vi "FVI_Manette_Process.vi"(2 "Axe R Y":dbl, 5 "Axe L Y":dbl, 6 "POV":dbl, 7 "Axe R X":dbl, 9 "Rtrigger":dbl, 11 "Axe L X":dbl) -> (1 "Correction angle":dbl, 4 "SwerveDrive":T1)   [LabVIEW 2018]
uses:
  SwerveDrive.ctl
  MyGlobal.vi
panel:
  in  "TD_SwerveDrive":T1
  out "arctan(x)":dbl
  out "x/y":dbl
  out "y < 0":bool
  out "x < 0":bool
  out "error out":errorcluster
  in  "error in (no error)":errorcluster
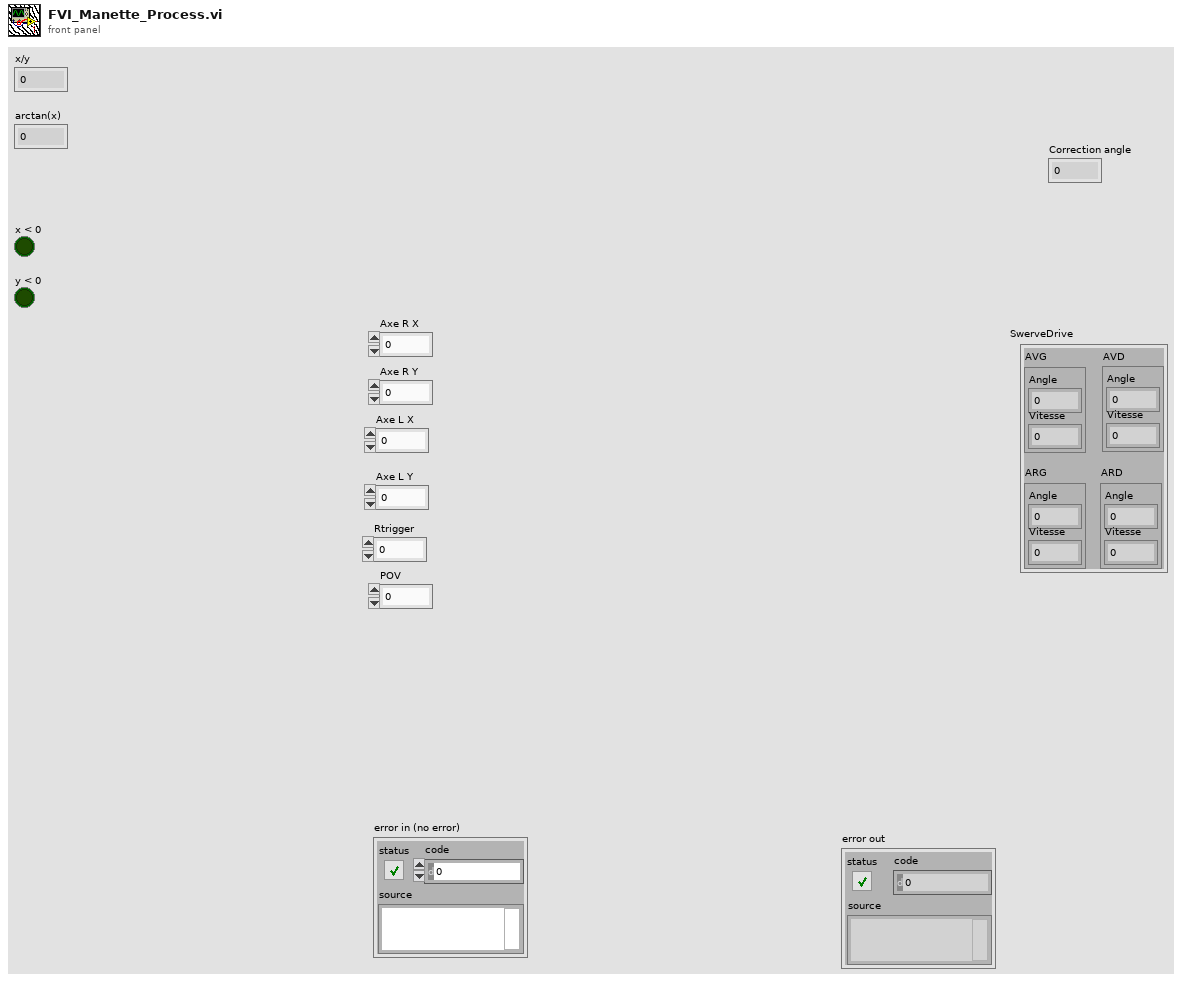
[diagram p1: front panel]
types:
  T1 = typedef "SwerveDrive.ctl" = cluster{"AVD":cluster{"Angle":dbl, "Vitesse":dbl}, "AVG":cluster{"Angle":dbl, "Vitesse":dbl}, "ARG":cluster{"Angle":dbl, "Vitesse":dbl}, "ARD":cluster{"Angle":dbl, "Vitesse":dbl}}
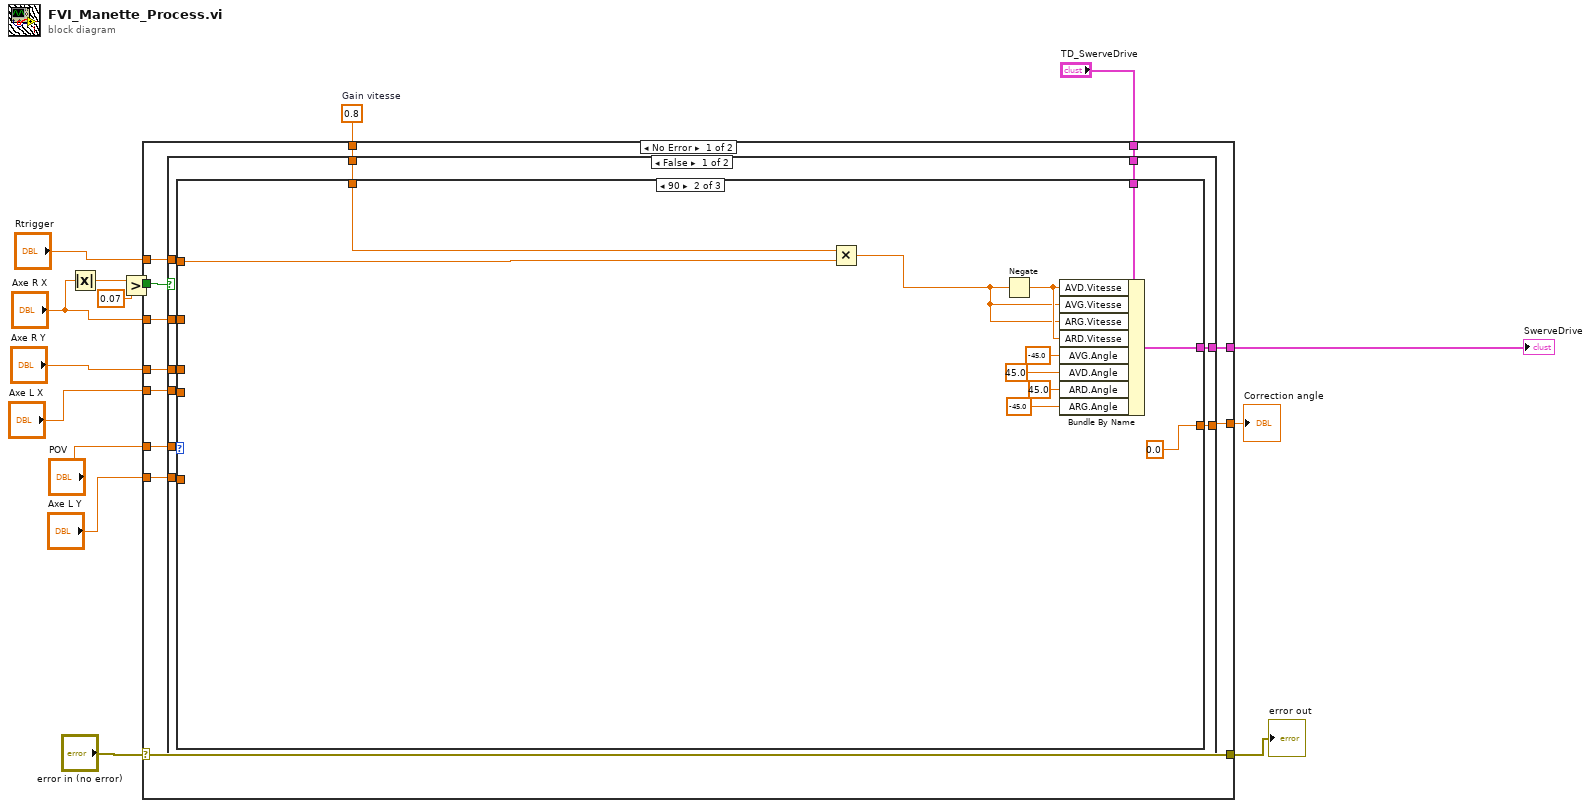
[diagram p0: block diagram]
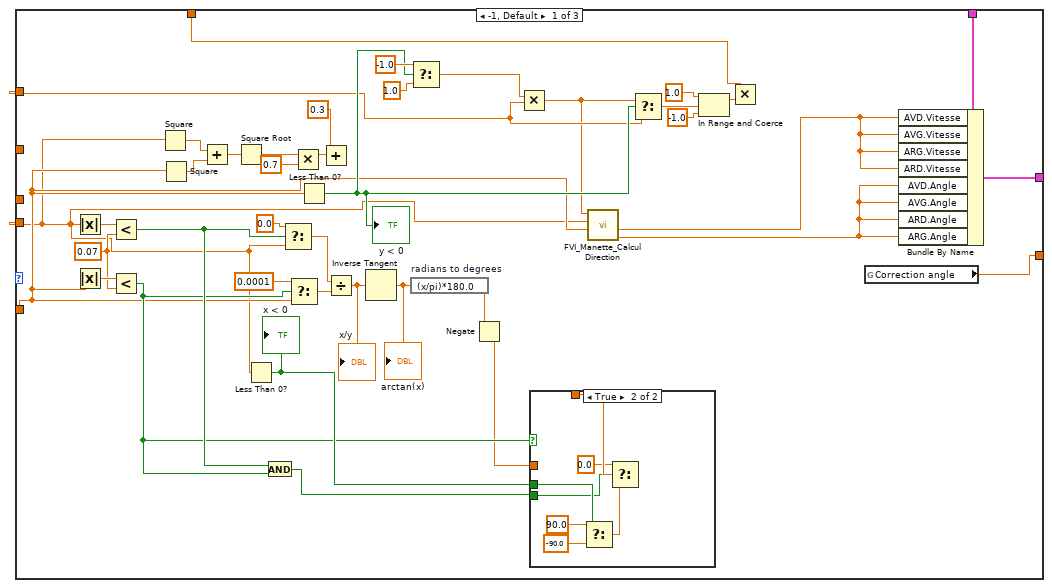
[diagram p2: hidden frame]
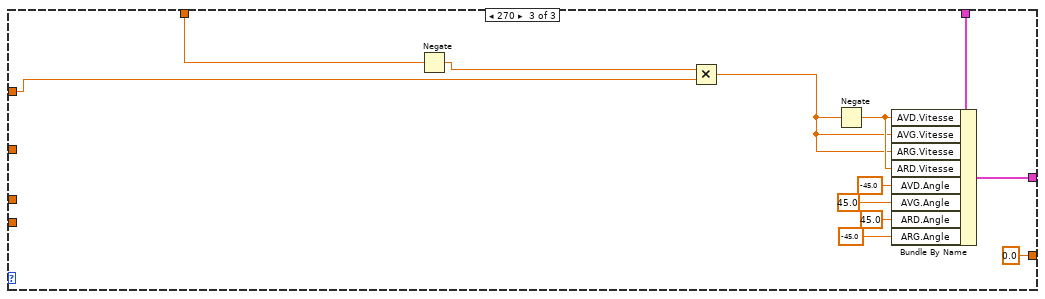
[diagram p4: hidden frame]
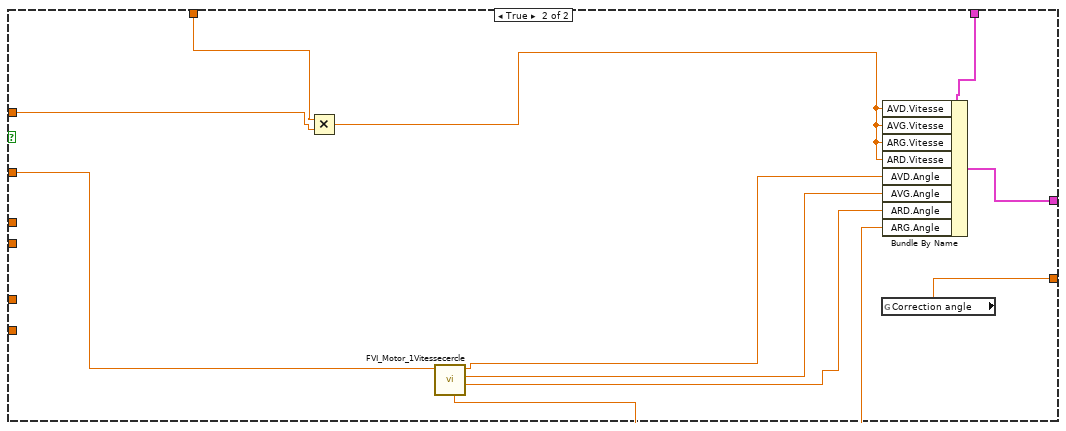
[diagram p5: hidden frame]
diagram:
  w5 = 0.8  # Gain vitesse
  n1 = Absolute Value(x="Axe R X") -> (abs(x)=w10:dbl)
  n2 = Greater?(x=w10, y=0.07 ("t")) -> (0:w8:bool)
  n3 = case shown="No Error" "error in (no error)" {
    selector: "error in (no error)" -> [w26 w121]
    tunnel: "Axe L X" -> [w25 _]
    tunnel: "Axe L Y" -> [w24 _]
    tunnel: [w27 _] -> w1
    tunnel: [w26 w121] -> w13
    tunnel: "Rtrigger" -> [w23 _]
    tunnel: "POV" -> [w22 _]
    tunnel: "Axe R X" -> [w21 _]
    tunnel: "Axe R Y" -> [w20 _]
    tunnel: w8 -> [w19 _]
    tunnel: w5 -> [w18 _]
    tunnel: "TD_SwerveDrive" -> [w17 w120]
    tunnel: [w16 w120] -> w2
    frame No Error {
      n4 = case shown="False" w19 {
        tunnel: [w28 w109] -> w27
        tunnel: w25 -> [w37 _]
        tunnel: w24 -> [w36 _]
        tunnel: w23 -> [w35 w119]
        tunnel: w22 -> [w34 _]
        tunnel: w21 -> [w33 w117]
        tunnel: w20 -> [w32 _]
        tunnel: w18 -> [w31 w118]
        tunnel: w17 -> [w30 w115]
        tunnel: [w29 w114] -> w16
        frame False {
          n5 = case shown="90" w34 {
            tunnel: w37 -> [w41 _ _]
            tunnel: w36 -> [w42 _ _]
            tunnel: w35 -> [w49 w96 w108]
            tunnel: w33 -> [_ _ _]
            tunnel: w32 -> [_ _ _]
            tunnel: w31 -> [w44 w95 w107]
            tunnel: w30 -> [w46 w94 w100]
            tunnel: [w45 w93 w99] -> w29
            tunnel: [w38 0.0 ("Correctiobn angle") 0.0 ("Correctiobn angle")] -> w28
            frame -1, Default {
              w67 = 0.07 ("t")
              n6 = Absolute Value(x=w41) -> (abs(x)=w76:dbl)
              n7 = Absolute Value(x=w42) -> (abs(x)=w77:dbl)
              n8 = Less?(x=w76, y=w67) -> (x < y?=w58:bool)
              n9 = Less?(x=w77, y=w67) -> (x < y?=w57:bool)
              n10 = Square(x=w41) -> (x^2=w54:dbl)
              n11 = Square(x=w42) -> (x^2=w55:dbl)
              n12 = Add(x=w54, y=w55) -> (x+y=w56:dbl)
              n13 = Square Root(x=w56) -> (sqrt(x)=w53:dbl)
              n14 = Less Than 0?(x=w41) -> (x < 0?=w71:bool)
              "x < 0" <- w71
              n15 = And(x=w58, y=w57) -> (x .and. y?=w75:bool)
              n16 = Select(t=0.0, s=w58, f=w41) -> (s? t:f=w63:dbl)
              n17 = Select(t=0.0001, s=w57, f=w42) -> (s? t:f=w61:dbl)
              n18 = Multiply(x=w53, y=0.7) -> (x*y=w51:dbl)
              n19 = Less Than 0?(x=w42) -> (x < 0?=w72:bool)
              "y < 0" <- w72
              n20 = Add(x=0.3, y=w51) -> ()  [unwired: 1 out]
              n21 = Divide(x=w63, y=w61) -> (x/y=w59:dbl)
              "x/y" <- w59
              n22 = Inverse Tangent(1:w59) -> (0:w60:dbl)
              "arctan(x)" <- w60
              n23 = Select(t=-1.0, s=w72, f=1.0) -> (s? t:f=w48:dbl)
              n24 = expression code="(x/pi)*180.0" "radians to degrees"(w60) -> (w69:dbl)
              n25 = Negate(x=w69) -> (-x=w47:dbl)
              n26 = Multiply(x=w48, y=w49) -> (x*y=w40:dbl)
              n27 = case shown="True" w57 {
                tunnel: w47 -> [w78 _]
                tunnel: w71 -> [_ w85]
                tunnel: [w78 w81] -> _
                tunnel: w75 -> [_ w79]
                frame False {
                }
                frame True {
                  n28 = Select(t=90.0, s=w85, f=-90.0) -> (s? t:f=w82:dbl)
                  n29 = Select(t=0.0, s=w79, f=w82) -> (s? t:f=w81:dbl)
                }
              }
              n30 = call "FVI_Manette_Calcul Direction.vi"("Axe L Y"=w42, "Axe L X"=w41, "Gain"=w40) -> ("Angle"=w39:dbl, "Vitesse"=w43:dbl)  [unwired: 5 in, 2 out]
              n31 = Select(t=w40, s=w72, f=w49) -> (s? t:f=w64:dbl)
              n32 = In Range and Coerce(upper limit=1.0 ("output high"), x=w64, lower limit=-1.0 ("output low")) -> (coerced(x)=w68:dbl)  [unwired: 1 out]
              n33 = Multiply(x=w44, y=w68) -> ()  [unwired: 1 out]
              n34 = global read "MyGlobal.vi" "Correction angle"() -> (w38:dbl)
              n35 = Bundle By Name(cluster=w46, "AVD.Vitesse"=w43, "AVG.Vitesse"=w43, "ARG.Vitesse"=w43, "ARD.Vitesse"=w43, "AVD.Angle"=w39, "AVG.Angle"=w39, "ARD.Angle"=w39, "ARG.Angle"=w39) -> (w45:T1)
            }
            frame 90 {
              n36 = Multiply(x=w95, y=w96) -> (x*y=w87:dbl)
              n37 = Negate(x=w87) -> (-x=w88:dbl)
              n38 = Bundle By Name(cluster=w94, "AVD.Vitesse"=w88, "AVG.Vitesse"=w87, "ARG.Vitesse"=w87, "ARD.Vitesse"=w88, "AVG.Angle"=-45.0 ("AVD.Angle"), "AVD.Angle"=45.0 ("AVG.Angle"), "ARD.Angle"=45.0, "ARG.Angle"=-45.0) -> (w93:T1)
            }
            frame 270 {
              n39 = Negate(x=w107) -> (-x=w106:dbl)
              n40 = Multiply(x=w106, y=w108) -> (x*y=w98:dbl)
              n41 = Negate(x=w98) -> (-x=w101:dbl)
              n42 = Bundle By Name(cluster=w100, "AVD.Vitesse"=w101, "AVG.Vitesse"=w98, "ARG.Vitesse"=w98, "ARD.Vitesse"=w101, "AVD.Angle"=-45.0, "AVG.Angle"=45.0, "ARD.Angle"=45.0, "ARG.Angle"=-45.0) -> (w99:T1)
            }
          }
        }
        frame True {
          n43 = Multiply(x=w118, y=w119) -> (x*y=w116:dbl)
          n44 = call "FVI_Motor_1Vitessecercle.vi"("Axe R X"=w117) -> ("ARD"=w111:dbl, "AVG"=w112:dbl, "AVD"=w113:dbl, "ARG"=w110:dbl)  [unwired: 7 in]
          n45 = global read "MyGlobal.vi" "Correction angle"() -> (w109:dbl)
          n46 = Bundle By Name(cluster=w115, "AVD.Vitesse"=w116, "AVG.Vitesse"=w116, "ARG.Vitesse"=w116, "ARD.Vitesse"=w116, "AVD.Angle"=w113, "AVG.Angle"=w112, "ARD.Angle"=w111, "ARG.Angle"=w110) -> (w114:T1)
        }
      }
    }
    frame Error {
    }
  }
  "error out" <- w13
  "SwerveDrive" <- w2
  "Correction angle" <- w1
